vi "Array processor.vi"(10 "Source array":bool[][](array[boolean]), 11 "Iterations":i32) -> (2 "Lenght product array":i32[][](array[numeric]), 3 "T/F product array":bool[][](array[boolean]))   [LabVIEW 2016]
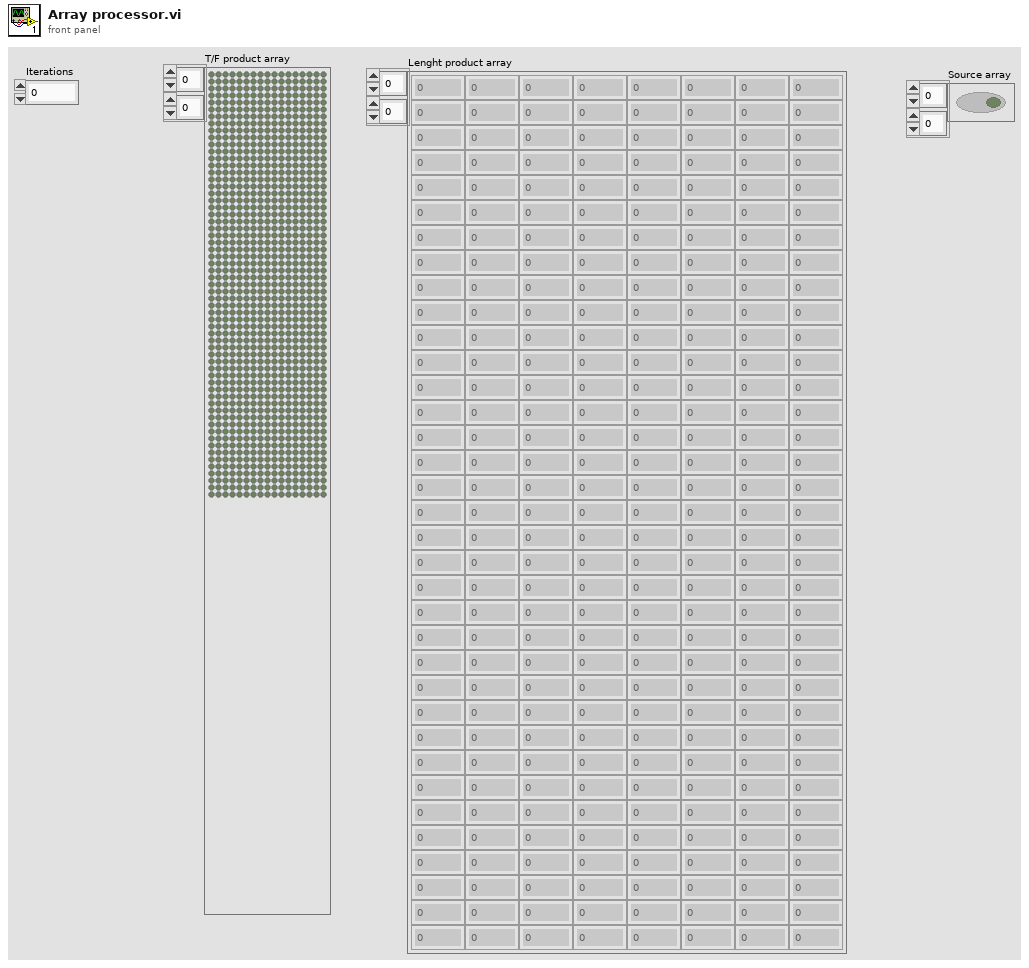
[diagram p1: front panel]
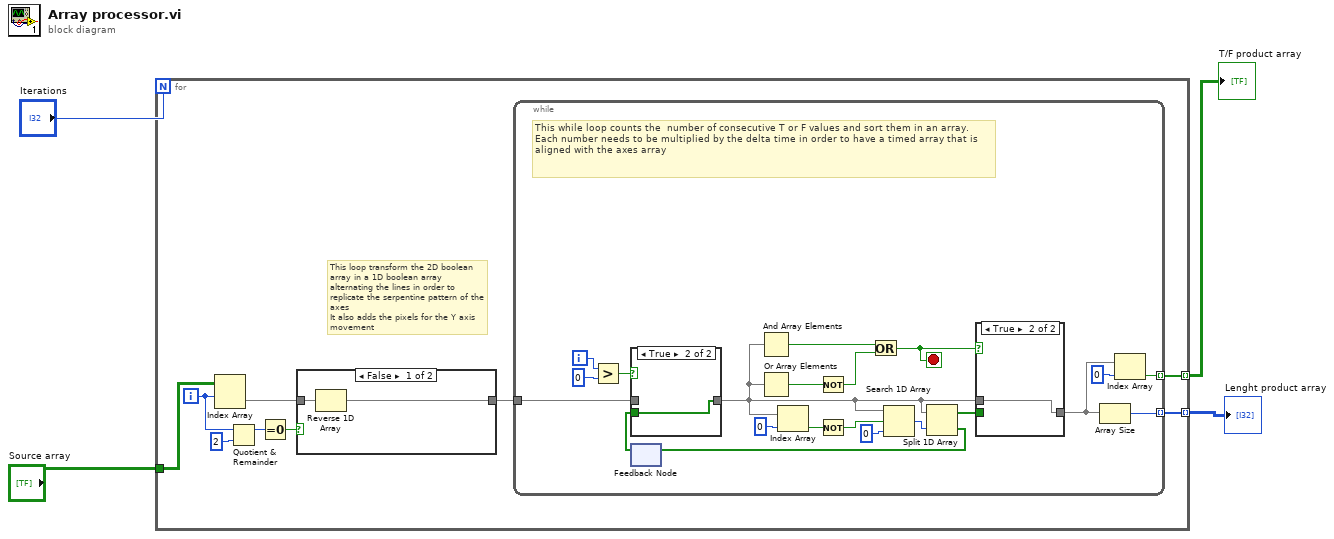
[diagram p0: block diagram]
diagram:
  n1 = for {
    N: "Iterations" -> [_]
    tunnel: "Source array" -> [w8]
    tunnel: [w6] -> w3 mode=indexing
    tunnel: [w5] -> w4 mode=indexing
    i -> [w11]
    # "This loop transform the 2D boolean array in a 1D boolean array alternating the lines in order to replicate the serpentine pattern of the axes\nIt also adds the pixels for the Y axis movement"
    n2 = Index Array(array=w8, index (row)=w11) -> (element=w9:bool[])  [unwired: 1 in]
    n3 = Quotient & Remainder(x=w11, y=2) -> (x-y*floor(x/y)=w13:i32)  [unwired: 1 out]
    n4 = Equal To 0?(x=w13) -> (x = 0?=w10:bool)
    n5 = case shown="False" w10 {
      tunnel: w9 -> [w40 w41]
      tunnel: [w39 w41] -> w7
      frame False {
        n6 = Reverse 1D Array(array=w40) -> (reversed array=w39:bool[])
      }
      frame True {
      }
    }
    n7 = while {
      tunnel: w7 -> [w28]
      tunnel: [w33] -> w6 mode=indexing
      tunnel: [w14] -> w5 mode=indexing
      i -> [w25]
      stop <- w17 stop-if-true
      # "This while loop counts the  number of consecutive T or F values and sort them in an array. Each number needs to be multiplied by the delta time in order to have a timed array that is aligned with the axes array"
      n8 = Greater?(x=w25, y=0) -> (0:w26:bool)
      n9 = feedback #1() -> (w27:bool[])  [unwired: 1 in]
      n10 = case shown="True" w26 {
        tunnel: w28 -> [w37 _]
        tunnel: [w37 w38] -> w18
        tunnel: w27 -> [_ w38]
        frame False {
        }
        frame True {
        }
      }
      n11 = And Array Elements(Boolean array=w18) -> (logical AND=w22:bool)
      n12 = Or Array Elements(Boolean array=w18) -> (logical OR=w20:bool)
      n13 = Index Array(array=w18, index=0) -> (element=w31:bool)
      n14 = Not(x=w20) -> (.not. x?=w19:bool)
      n15 = Not(x=w31) -> (.not. x?=w30:bool)
      n16 = Or(x=w22, y=w19) -> (x .or. y?=w17:bool)
      n17 = Search 1D Array(1D array=w18, element=w30, start index (0)=0) -> (index of element=w29:i32)
      n18 = Split 1D Array(array=w18, index=w29) -> (first subarray=w21:bool[], second subarray=w23:bool[])
      n19 = feedback-in #1(w23) -> ()
      n20 = case shown="True" w17 {
        tunnel: w21 -> [w35 _]
        tunnel: [w35 w36] -> w16
        tunnel: w18 -> [_ w36]
        frame False {
        }
        frame True {
        }
      }
      n21 = Array Size(array=w16) -> (size(s)=w33:i32)
      n22 = Index Array(array=w16, index=0) -> (element=w14:bool)
    }
  }
  "T/F product array" <- w4
  "Lenght product array" <- w3
